vi "GetName.vi"(8 "error in (no error)":errorcluster, 11 "Pizza in":refnum<class "Pizza.lvclass">) -> (0 "error out":errorcluster, 2 "Name":string, 3 "Pizza out":refnum<class "Pizza.lvclass">)   [LabVIEW 2020, in "FactoryMethod.lvlib" / "PizzaFactoryMethod.lvlib" / "Pizza.lvclass"]
uses:
  Pizza.lvclass
  Pizza.lvclass/Pizza.ctl
  Private/Property/name/Read name.vi
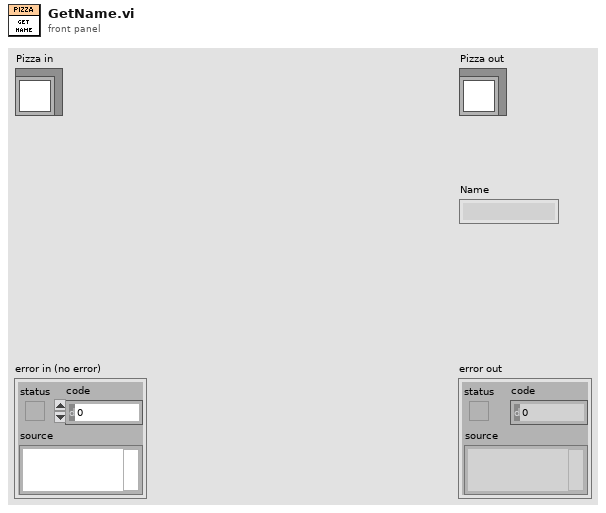
[diagram p1: front panel]
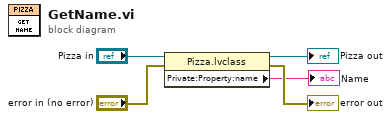
[diagram p0: block diagram]
diagram:
  n1 = property class="Pizza.lvclass"(reference="Pizza in", error in="error in (no error)") -> (reference out=→"Pizza out":refnum<class "Pizza.lvclass">, error out=→"error out":errorcluster, "Private:Property:name"=→"Name":string)
